vi "ReadChangedFileLogPaths.vi"(8 "error in (no error)":errorcluster, 10 "Workspace Path":path, 11 "Refnum in":T1) -> (0 "error out":errorcluster, 2 "ChangedFilesLogpaths":map{string, path}(c390), 3 "refnum out":T1)   [LabVIEW 2019, in "DepsWatch.lvlib"]
uses:
  DepsWatch.lvlib
  <vilib>/Utility/config.llb/Config Data RefNum.ctl
  <vilib>/Utility/config.llb/Read Key (String).vi
  <vilib>/Utility/config.llb/NI_LVConfig.lvlib
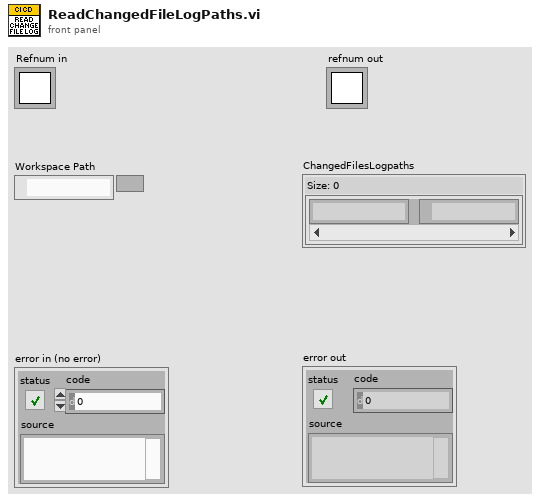
[diagram p1: front panel]
types:
  T1 = typedef "NI_LVConfig.lvlib/Config Data RefNum.ctl" = refnum<k1>
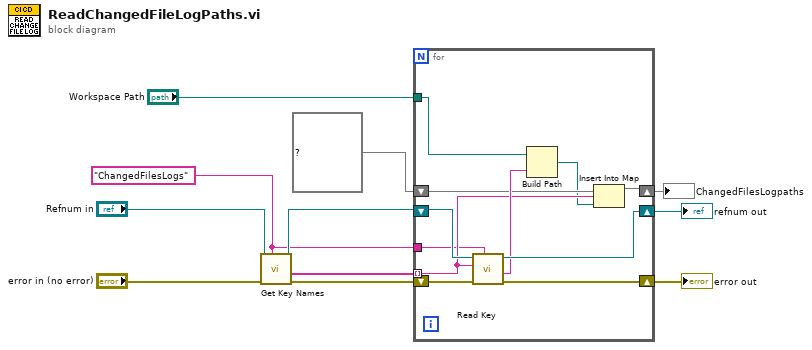
[diagram p0: block diagram]
diagram:
  w1 = "ChangedFilesLogs" ("section")
  n1 = call <vilib>:"Get Key Names.vi"("section"=w1, "error in (no error)"="error in (no error)", "refnum"="Refnum in") -> ("error out"=w9:errorcluster, "key names"=w10:string[], "refnum out"=w8:T1)  [unwired: 5 in, 1 out]
  n2 = for {
    shift-right: [w20] -> w4
    shift-left: w9 -> [w20]
    tunnel: w10 -> [w15] mode=indexing
    tunnel: "Workspace Path" -> [w21]
    shift-right: [w18] -> w5
    shift-left: w8 -> [w19]
    shift-right: [w13] -> w2
    shift-left: map{string, path} {} ("map") -> [w16]
    tunnel: w1 -> [w12]
    n3 = call-poly <vilib>:"Read Key.vi"("section"=w12, "error in (no error)"=w20, "key"=w15, "refnum"=w19) -> ("value"=w17:string, "refnum out"=w18:T1)  [unwired: 4 in, 2 out]
    n4 = Build Path(base path=w21, name or relative path=w17) -> (appended path=w14:path)
    n5 = Insert Into Map(map in=w16, key=w15, value=w14) -> (map out=w13:map{string, path})  [unwired: 2 out]
  }
  "refnum out" <- w5
  "error out" <- w4
  "ChangedFilesLogpaths" <- w2
